vi "get channels.vi"(11 "user tag bus module configuration In":refnum<class "user tag bus module configuration.lvclass">) -> (2 "channels":refnum<class "TBM channel.lvclass">[](array[class]), 3 "user tag bus module configuration Out":refnum<class "user tag bus module configuration.lvclass">)   [LabVIEW 2013, in "user tag bus module configuration.lvclass"]
uses:
  user tag bus module configuration.lvclass
  <vilib>/NI/Tag Bus Module Framework/channel/TBM channel.lvclass
  user tag bus module configuration.lvclass/user tag bus module configuration.ctl
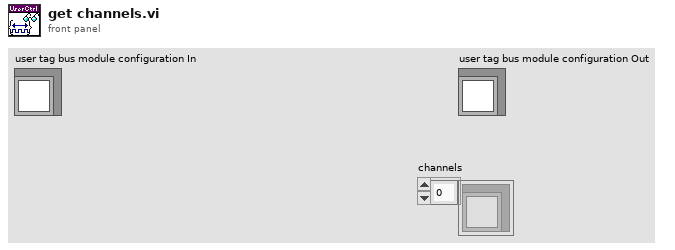
[diagram p1: front panel]
types:
  T1 = typedef "user tag bus module configuration.lvclass/state module configuration.ctl" = cluster{"fixed input":refnum<class "TBM channel.lvclass">, "fixed output":refnum<class "TBM channel.lvclass">, "initial state":u8}
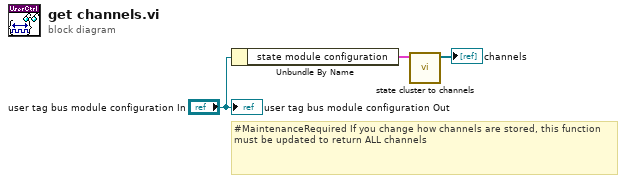
[diagram p0: block diagram]
diagram:
  # "#MaintenanceRequired If you change how channels are stored, this function must be updated to return ALL channels"
  n1 = Unbundle By Name("user tag bus module configuration In") -> ("state module configuration"=w2:T1)
  n2 = call "state cluster to channels.vi"("state module configuration"=w2) -> ("channels"=→"channels":refnum<class "TBM channel.lvclass">[])  [unwired: 10 in]
  "user tag bus module configuration Out" <- "user tag bus module configuration In"
